vi "Configure Serial Channel Display Parameters.vi"(0 "fpga interface in":refnum<k20>, 5 "serial channel configurations":T1[](array[typedef]) {"RAW Display Parameters"."Bayer Parameters"."Blue Gain" format="%_4g"; "RAW Display Parameters"."Bayer Parameters"."Green Gain" format="%_4g"; "RAW Display Parameters"."Bayer Parameters"."Red Gain" format="%_4g"; "RAW Display Parameters"."Bayer Parameters"."Algorithm" items=["Bilinear", "VNG"]; "RAW Display Parameters"."Bayer Parameters"."Pattern" items=["GB", "GR", "BG", "RG"]}, 11 "error in (no error)":errorcluster) -> (4 "fpga interface out":refnum<k20>, 6 "serial channel display parameters":T5[](array[typedef]) {"RAW parameters"."bayer parameters"."blue gain" format="%_4g"; "RAW parameters"."bayer parameters"."green gain" format="%_4g"; "RAW parameters"."bayer parameters"."red gain" format="%_4g"; "RAW parameters"."bayer parameters"."algorithm" items=["Bilinear", "VNG"]; "RAW parameters"."bayer parameters"."pattern" items=["GB", "GR", "BG", "RG"]}, 8 "serial channels":string[](array[string]), 15 "error out":errorcluster)   [LabVIEW 2023, in "GettingStarted_Common_148X_Host.lvlib"]
uses:
  GettingStarted_Common_148X_Host.lvlib
  Types/Serial Channel Display Parameters.ctl
  <vilib>/vision/Image Controls.llb/IMAQ Image.ctl
  Types/RAW Interpretation for Display.ctl
  Types/Serial Channel Configuration.ctl
  <instrlib>/FlexRIO/CSI-2/v2/FPGA/Types/Display Parameters.ctl
  <instrlib>/FlexRIO/CSI-2/v2/Common/Types/LLP Data Type.ctl
  Types/148x_Common_FPGA_Reference.ctl
  3fe83519-f268-4271-b3b5-7a670f563992.vi
  <vilib>/rvi/errors/niLvFpgaAdjustHostInterfaceError.vi
  <vilib>/rvi/interface/nirviReadWriteControl/nirviReadWriteControl.xnode
  <instrlib>/FlexRIO/Automotive Vision Utility/v1/Host/Automotive Vision Utility.lvlib
  <instrlib>/FlexRIO/CSI-2/v2/FPGA/NI CSI-2 API FPGA v2.lvlib
  NiFpgaLv.dll
  <vilib>/rvi/interface/Simulation/niFpgaSimulationCallBeginRW.vi
  <instrlib>/FlexRIO/CSI-2/v2/Common/NI CSI-2 API Common v2.lvlib
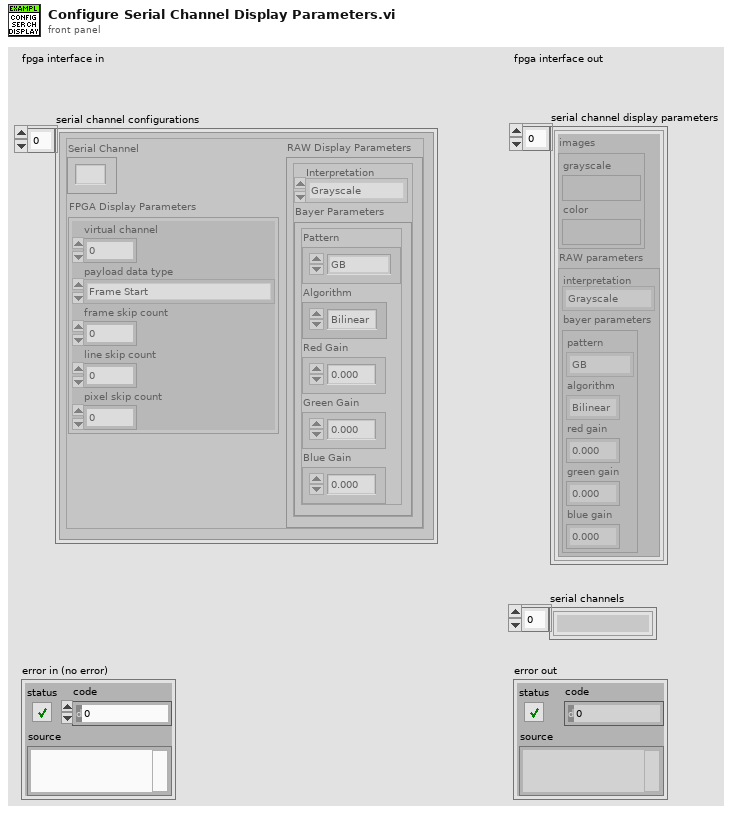
[diagram p1: front panel]
types:
  T1 = typedef "GettingStarted_Common_148X_Host.lvlib/Serial Channel Configuration.ctl" = cluster{"Serial Channel":string, "FPGA Display Parameters":T2, "RAW Display Parameters":cluster{"Interpretation":T4, "Bayer Parameters":cluster{"Pattern":i32, "Algorithm":i32, "Red Gain":dbl, "Green Gain":dbl, "Blue Gain":dbl}}}
  T2 = typedef "NI CSI-2 API FPGA v2.lvlib/Display Parameters.ctl" = cluster{"virtual channel":fxp<+,4,4>, "payload data type":T3, "frame skip count":u16, "line skip count":u8, "pixel skip count":fxp<+,5,5>}
  T3 = typedef "NI CSI-2 API Common v2.lvlib/LLP Data Type.ctl" = enum8{"Frame Start", "Frame End", "Line Start", "Line End", "End of Transmission", "Reserved 0", "Reserved 1", "Reserved 2", "Generic Short Packet 1", "Generic Short Packet 2", "Generic Short Packet 3", "Generic Short Packet 4", "Generic Short Packet 5", "Generic Short Packet 6", "Generic Short Packet 7", "Generic Short Packet 8", "Null", "Blanking Data", "Embedded 8-bit non Image Data", "Generic Long Packet 1", "Generic Long Packet 2", "Generic Long Packet 3", "Generic Long Packet 4", "Reserved 3", "YUV420 8-bit", "YUV420 10-bit", "Legacy YUV420 8-bit", "Reserved 4", "YUV420 8-bit Chroma Shifted", "YUV420 10-bit Chroma Shifted", "YUV422 8-bit", "YUV422 10-bit", "RGB444", "RGB555", "RGB565", "RGB666", "RGB888", "Reserved 5", "Reserved 6", "RAW 24", "RAW 6", "RAW 7", "RAW 8", "RAW 10", "RAW 12", "RAW 14", "RAW 16", "RAW 20", "User Defined 8-bit Data 1", "User Defined 8-bit Data 2", "User Defined 8-bit Data 3", "User Defined 8-bit Data 4", "User Defined 8-bit Data 5", "User Defined 8-bit Data 6", "User Defined 8-bit Data 7", "User Defined 8-bit Data 8", "USL Command", "Reserved 7", "Reserved 8", "Reserved 9", "Reserved 10", "Reserved 11", "Reserved 12", "LRTE EPD Spacer"}
  T4 = typedef "GettingStarted_Common_148X_Host.lvlib/RAW Interpretation for Display.ctl" = enum16{"Grayscale", "Bayer", "RGB", "YUV422", "YUV420", "Legacy YUV420"}
  T5 = typedef "GettingStarted_Common_148X_Host.lvlib/Serial Channel Display Parameters.ctl" = cluster{"images":cluster{"grayscale":T6, "color":T6}, "RAW parameters":cluster{"interpretation":T4, "bayer parameters":cluster{"pattern":i32, "algorithm":i32, "red gain":dbl, "green gain":dbl, "blue gain":dbl}}}
  T6 = typedef "IMAQ Image.ctl" = refnum<image>
  T7 = typedef "GettingStarted_Common_148X_Host.lvlib/148x_Common_FPGA_Reference.ctl" = refnum<k20>
  T8 = cluster{"Interpretation":T4, "Bayer Parameters":cluster{"Pattern":i32, "Algorithm":i32, "Red Gain":dbl, "Green Gain":dbl, "Blue Gain":dbl}}
  T9 = typedef "Image Type" = u32
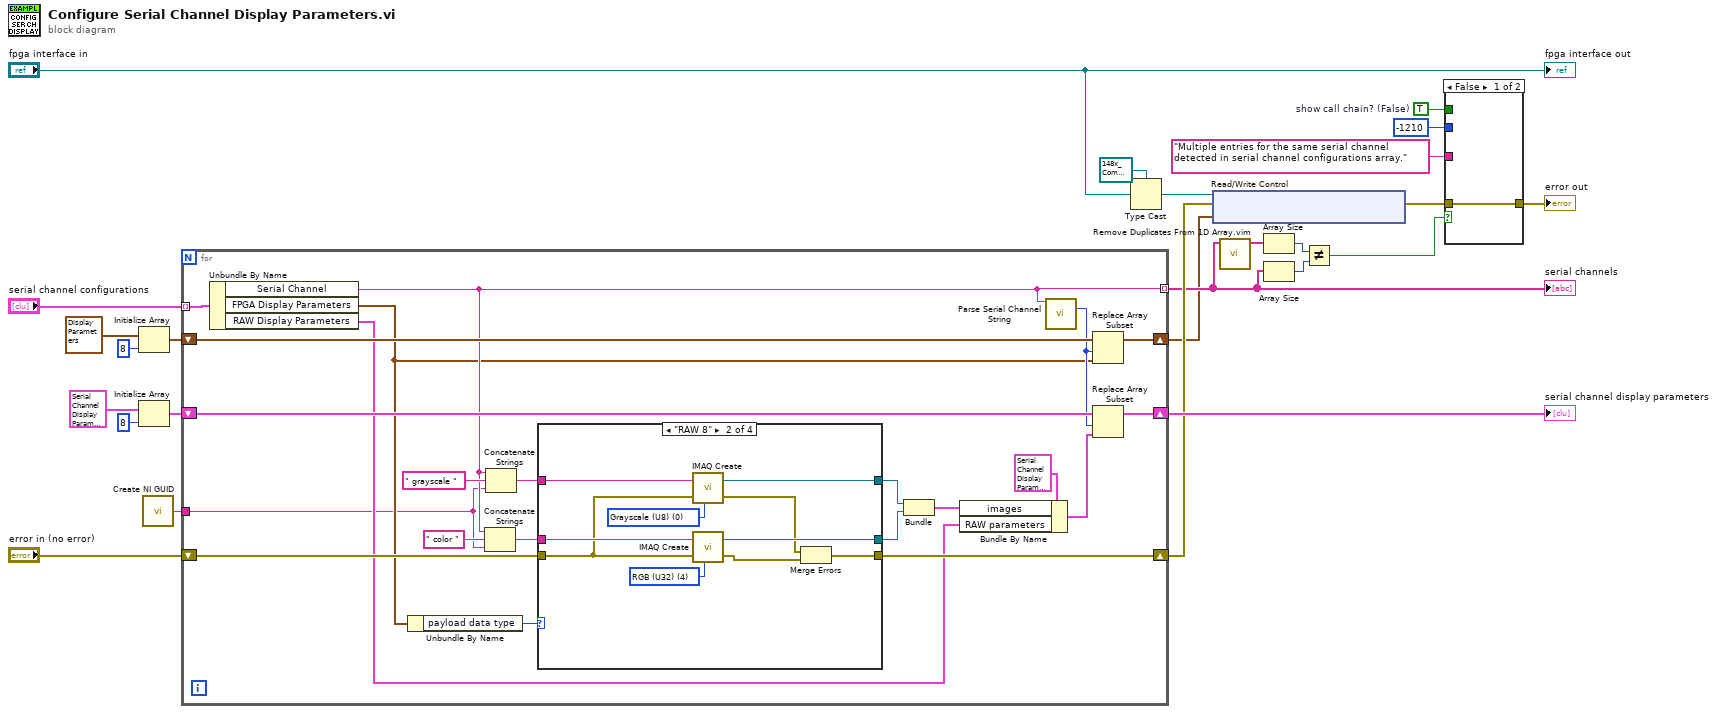
[diagram p0: block diagram]
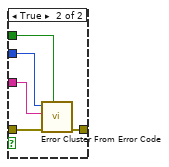
[diagram p2: hidden frame]
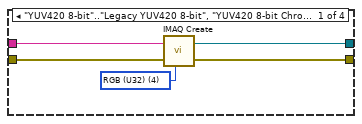
[diagram p3: hidden frame]
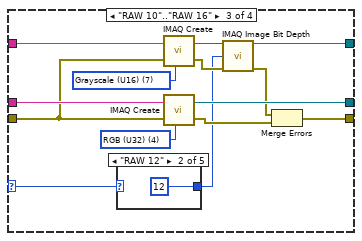
[diagram p4: hidden frame]
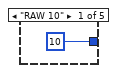
[diagram p5: hidden frame]
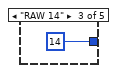
[diagram p6: hidden frame]
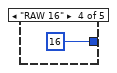
[diagram p7: hidden frame]
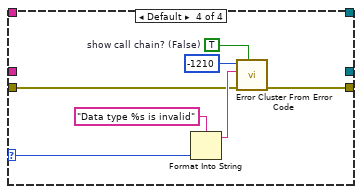
[diagram p9: hidden frame]
diagram:
  w7 = TRUE  # show call chain? (False)
  n1 = Initialize Array(T2 {"virtual channel"=0.0, "payload data type"=enum."Frame Start", "frame skip count"=0, "line skip count"=0, "pixel skip count"=0.0} ("fpga display parameters"), 8 ("dimension size")) -> (w19:T2[])
  n2 = Initialize Array(T5 {"images"={"grayscale"=refnum, "color"=refnum}, "RAW parameters"={"interpretation"=enum."Grayscale", "bayer parameters"={"pattern"=0, "algorithm"=0, "red gain"=1.0, "green gain"=1.0, "blue gain"=1.0}}} ("serial channel display parameters"), 8 ("dimension size")) -> (w18:T5[])
  n3 = call <vilib>:"Create NI GUID.vi"() -> ("NI GUID"=w1:string)
  n4 = for {
    shift-right: [w43] -> w2
    shift-left: w19 -> [w44]
    shift-right: [w45] -> w24
    shift-left: w18 -> [w46]
    tunnel: "serial channel configurations" -> [w47] mode=indexing
    tunnel: [w37] -> w11 mode=indexing
    shift-right: [w34] -> w23
    shift-left: "error in (no error)" -> [w35]
    tunnel: w1 -> [w26]
    n5 = Unbundle By Name(w47) -> ("Serial Channel"=w37:string, "FPGA Display Parameters"=w28:T2, "RAW Display Parameters"=w27:T8)
    n6 = Unbundle By Name(w28) -> ("payload data type"=w41:T3)
    n7 = Concatenate Strings(w37, " color " ("Image Name"), w26) -> (w36:string)
    n8 = Concatenate Strings(w37, " grayscale " ("Image Name"), w26) -> (w39:string)
    n9 = case shown="\"RAW 8\"" w41 {
      selector: w41 -> [_ _ w70 w84]
      tunnel: w39 -> [_ w62 w76 _]
      tunnel: w36 -> [w51 w61 w75 _]
      tunnel: w35 -> [w50 w60 w74 w82]
      tunnel: [w48 w59 w73 w81] -> w34
      tunnel: [w49 w58 w72 _] -> w31
      tunnel: [_ w57 w71 _] -> w32
      frame "YUV420 8-bit".."Legacy YUV420 8-bit", "YUV420 8-bit Chroma Shifted".."YUV422 10-bit", "RGB565".."RGB888" {
        w52 = T9 4 items=["Grayscale (U8)", "Grayscale (I16)", "Grayscale (SGL)", "Complex (CSG)", "RGB (U32)", "HSL (U32)", "RGB (U64)", "Grayscale (U16)"] ("Image Type")
        n10 = call "IMAQ Create"("Image Name"=w51, "Image Type"=w52, "error in (no error)"=w50) -> ("New Image"=w49:T6, "error out"=w48:errorcluster)  [unwired: 2 in]
      }
      frame "RAW 8" {
        w55 = T9 4 items=["Grayscale (U8)", "Grayscale (I16)", "Grayscale (SGL)", "Complex (CSG)", "RGB (U32)", "HSL (U32)", "RGB (U64)", "Grayscale (U16)"] ("Image Type")
        w56 = T9 0 items=["Grayscale (U8)", "Grayscale (I16)", "Grayscale (SGL)", "Complex (CSG)", "RGB (U32)", "HSL (U32)", "RGB (U64)", "Grayscale (U16)"] ("Image Type")
        n11 = call "IMAQ Create"("Image Name"=w62, "Image Type"=w56, "error in (no error)"=w60) -> ("New Image"=w57:T6, "error out"=w53:errorcluster)  [unwired: 2 in]
        n12 = call "IMAQ Create"("Image Name"=w61, "Image Type"=w55, "error in (no error)"=w60) -> ("New Image"=w58:T6, "error out"=w54:errorcluster)  [unwired: 2 in]
        n13 = Merge Errors(w53, w54) -> (w59:errorcluster)
      }
      frame "RAW 10".."RAW 16" {
        w68 = T9 4 items=["Grayscale (U8)", "Grayscale (I16)", "Grayscale (SGL)", "Complex (CSG)", "RGB (U32)", "HSL (U32)", "RGB (U64)", "Grayscale (U16)"] ("Image Type")
        w69 = T9 7 items=["Grayscale (U8)", "Grayscale (I16)", "Grayscale (SGL)", "Complex (CSG)", "RGB (U32)", "HSL (U32)", "RGB (U64)", "Grayscale (U16)"] ("Image Type")
        n14 = case shown="\"RAW 12\"" w70 {
          tunnel: [u32 10 ("Bit Depth (0)") u32 12 ("Bit Depth (0)") u32 14 ("Bit Depth (0)") u32 16 ("Bit Depth (0)") _] -> w63
          frame "RAW 10" {
          }
          frame "RAW 12" {
          }
          frame "RAW 14" {
          }
          frame "RAW 16" {
          }
          frame Default {
          }
        }
        n15 = call "IMAQ Create"("Image Name"=w76, "Image Type"=w69, "error in (no error)"=w74) -> ("New Image"=w66:T6, "error out"=w65:errorcluster)  [unwired: 2 in]
        n16 = call "IMAQ Create"("Image Name"=w75, "Image Type"=w68, "error in (no error)"=w74) -> ("New Image"=w72:T6, "error out"=w67:errorcluster)  [unwired: 2 in]
        n17 = call "IMAQ Image Bit Depth"("Image"=w66, "Bit Depth (0)"=w63, "error in (no error)"=w65) -> ("Image Out"=w71:T6, "error out"=w64:errorcluster)  [unwired: 10 in, 1 out]
        n18 = Merge Errors(w64, w67) -> (w73:errorcluster)
      }
      frame Default {
        w86 = TRUE  # show call chain? (False)
        n19 = Format Into String(format string="Data type %s is invalid" ("error message (\"\")"), w84) -> (resulting string=w83:string)  [unwired: 2 in, 1 out]
        n20 = call <vilib>:"Error Cluster From Error Code.vi"("show call chain? (False)"=w86, "error in (no error)"=w82, "error message (\"\")"=w83, "error code (0)"=-1210) -> ("error out"=w81:errorcluster)  [unwired: 5 in]
      }
    }
    n21 = Bundle("Image Out"=w32, "New Image"=w31) -> (w30:cluster{"Image Out":T6, "New Image":T6})  [unwired: 1 in]
    n22 = Bundle By Name(cluster=T5 {"images"={"grayscale"=refnum, "color"=refnum}, "RAW parameters"={"interpretation"=enum."Grayscale", "bayer parameters"={"pattern"=0, "algorithm"=0, "red gain"=1.0, "green gain"=1.0, "blue gain"=1.0}}} ("serial channel display parameters"), "images"=w30, "RAW parameters"=w27) -> (w29:T5)
    n23 = call <instrlib>:"Parse Serial Channel String.vi"("serial channel string"=w37) -> ("channel number"=w42:i32)  [unwired: 13 in, 1 out]
    n24 = Replace Array Subset(array=w44, new element=w28, index=w42) -> (w43:T2[])
    n25 = Replace Array Subset(array=w46, new element=w29, index=w42) -> (w45:T5[])
  }
  "serial channels" <- w11
  "serial channel display parameters" <- w24
  n26 = Type Cast(type=T7 refnum ("FPGA VI Reference Out"), x="fpga interface in") -> (*(type *) &x=w22:T7)
  n27 = xnode "Read/Write Control"("FPGA VI Reference In"=w22, "error in"=w23, "serial channel display parameters"=w2) -> ("error out"=w5:errorcluster)  [unwired: 1 out]
  n28 = call "Remove Duplicates From 1D Array.vim"("array"=w11) -> ("array with duplicates removed"=w12:string[])  [unwired: 10 in]
  n29 = Array Size(array=w12) -> (size(s)=w10:i32)
  n30 = Array Size(array=w11) -> (size(s)=w9:i32)
  n31 = Not Equal?(x=w10, y=w9) -> (x != y?=w4:bool)
  n32 = case shown="False" w4 {
    tunnel: -1210 ("error code (0)") -> [_ w93]
    tunnel: w7 -> [_ w92]
    tunnel: "Multiple entries for the same serial channel detected in serial channel configurations array." ("error message (\"\")") -> [_ w91]
    tunnel: [w88 w90] -> w6
    tunnel: w5 -> [w88 w89]
    frame False {
    }
    frame True {
      n33 = call <vilib>:"Error Cluster From Error Code.vi"("show call chain? (False)"=w92, "error in (no error)"=w89, "error message (\"\")"=w91, "error code (0)"=w93) -> ("error out"=w90:errorcluster)  [unwired: 5 in]
    }
  }
  "error out" <- w6
  "fpga interface out" <- "fpga interface in"
